vi "Refname to String (Sensors).vi"(1 "Enum":T1) -> (0 "String":string)   [LabVIEW 2016]
uses:
  Sensors.ctl
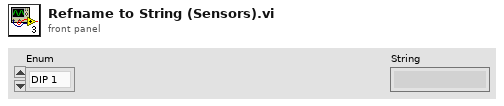
[diagram p1: front panel]
types:
  T1 = typedef "Sensors.ctl" = enum16{"DIP 1", "DIP 2", "DIP 3", "DIP 4"}
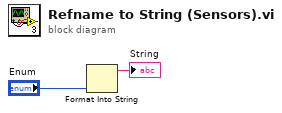
[diagram p0: block diagram]
diagram:
  n1 = Format Into String("Enum") -> (resulting string=→"String":string)  [unwired: 3 in, 1 out]
